vi "Generator Drive RTD offset.vi"(0 "RTD1 Offset 1":dbl, 1 "RTD2 Offset":dbl, 2 "RTD3 Offset":dbl, 3 "RTD4 Offset":dbl, 4 "RTD5 Offset":dbl, 5 "RTD6 Offset":dbl, 7 "V ref":dbl, 8 "Write/Read":enum16{"Write", "Read"}(ring)=enum."Read") -> (13 "V ref":dbl, 14 "RTD1 Offset Out":dbl, 15 "RTD2 Offset Out":dbl, 16 "RTD3 Offset Out":dbl, 17 "RTD4 Offset out":dbl, 18 "RTD5 Offset out":dbl, 19 "RTD6 Offset  out":dbl)   [LabVIEW 2022 SP3]
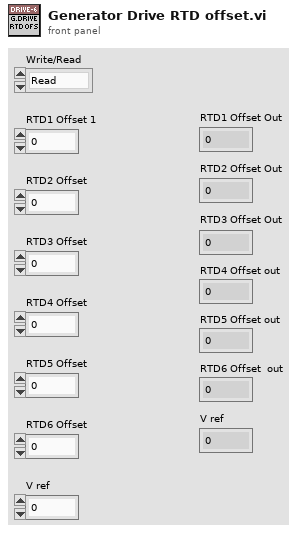
[diagram p1: front panel]
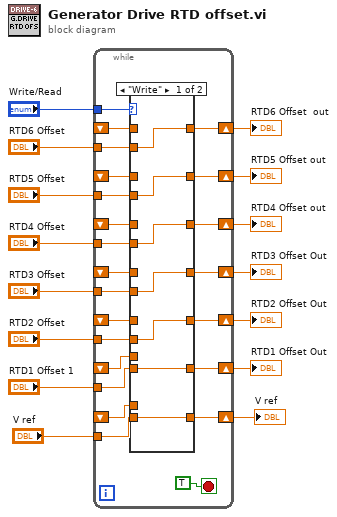
[diagram p0: block diagram]
diagram:
  n1 = while {
    shift-right: [w37] -> w13
    shift-left: _ -> [w35]
    tunnel: "Write/Read" -> [w38]
    tunnel: "RTD1 Offset 1" -> [w36]
    tunnel: "RTD2 Offset" -> [w33]
    shift-right: [w32] -> w11
    shift-left: _ -> [w31]
    tunnel: "RTD3 Offset" -> [w30]
    shift-right: [w29] -> w9
    shift-left: _ -> [w28]
    tunnel: "RTD4 Offset" -> [w27]
    tunnel: "RTD5 Offset" -> [w26]
    tunnel: "RTD6 Offset" -> [w25]
    shift-right: [w24] -> w5
    shift-left: _ -> [w21]
    shift-right: [w23] -> w4
    shift-left: _ -> [w20]
    shift-right: [w22] -> w3
    shift-left: _ -> [w19]
    shift-right: [w16] -> w2
    shift-left: _ -> [w18]
    tunnel: "V ref" -> [w17]
    stop <- TRUE stop-if-true
    n2 = case shown="\"Write\"" w38 {
      tunnel: w36 -> [w45 _]
      tunnel: [w45 w52] -> w37
      tunnel: w35 -> [_ w52]
      tunnel: w33 -> [w44 _]
      tunnel: [w44 w51] -> w32
      tunnel: w31 -> [_ w51]
      tunnel: w30 -> [w43 _]
      tunnel: [w43 w50] -> w29
      tunnel: w28 -> [_ w50]
      tunnel: w27 -> [w42 _]
      tunnel: w26 -> [w41 _]
      tunnel: w25 -> [w40 _]
      tunnel: [w42 w49] -> w24
      tunnel: [w41 w48] -> w23
      tunnel: [w40 w47] -> w22
      tunnel: w21 -> [_ w49]
      tunnel: w20 -> [_ w48]
      tunnel: w19 -> [_ w47]
      tunnel: w17 -> [w39 _]
      tunnel: [w39 w46] -> w16
      tunnel: w18 -> [_ w46]
      frame "Write" {
      }
      frame "Read", Default {
      }
    }
  }
  "RTD1 Offset Out" <- w13
  "RTD2 Offset Out" <- w11
  "RTD3 Offset Out" <- w9
  "RTD4 Offset out" <- w5
  "RTD5 Offset out" <- w4
  "RTD6 Offset  out" <- w3
  "V ref" <- w2
